vi "U6 Multiple LJTDAC Loop.vi"() -> (0 "error out":errorcluster)   [LabVIEW 2021]
panel:
  in  "Interval (ms)":u32=500
  in  "stop":bool
  in  "2nd DACB":dbl step=0.1 format="%.4f"
  in  "2nd DACA":dbl step=0.1 format="%.4f"
  in  "2nd TDAC SCL Pin #":i32=2
  in  "1st DACB":dbl step=0.1 format="%.4f"
  in  "1st DACA":dbl step=0.1 format="%.4f"
  in  "FirstFound":bool=TRUE
  in  "Address":string="1"
  out "Error Message":string
  in  "1st TDAC SCL Pin #":i32
  # "Updates both channels on an LJTick-DAC."
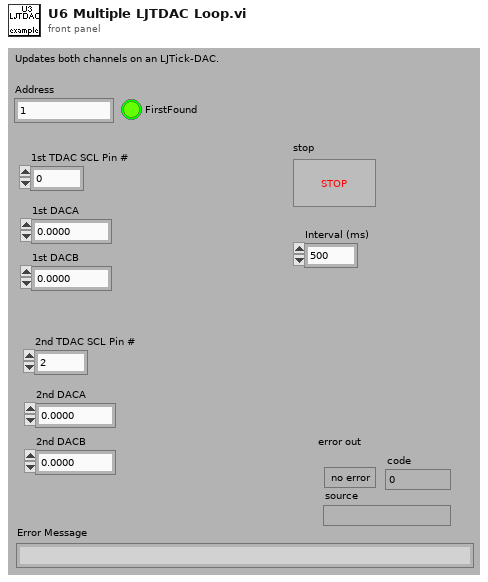
[diagram p1: front panel]
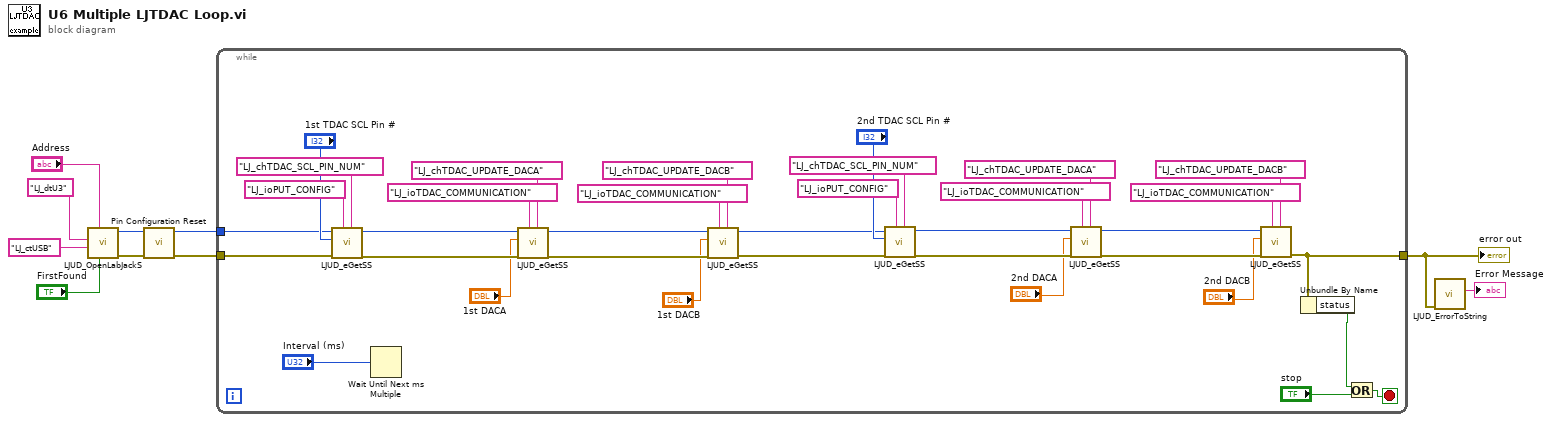
[diagram p0: block diagram]
diagram:
  n1 = call "LJUD_OpenLabJackS.vi"("FirstFound"="FirstFound", "Address"="Address", "ConnectionType"="LJ_ctUSB", "DeviceType"="LJ_dtU3") -> ("error out"=w4:errorcluster, "Handle"=w5:i32)  [unwired: 5 in, 1 out]
  n2 = call "Pin Configuration Reset.vi"("error in"=w4, "Handle In"=w5) -> ("error out"=w2:errorcluster, "Handle Out"=w3:i32)  [unwired: 8 in]
  n3 = while {
    tunnel: w3 -> [w42]
    tunnel: w2 -> [w41]
    tunnel: [w11] -> w1
    stop <- w16 stop-if-true
    n4 = call "LJUD_eGetSS.vi"("Channel"="LJ_chTDAC_SCL_PIN_NUM", "IOType"="LJ_ioPUT_CONFIG", "error in"=w41, "Value Write"="1st TDAC SCL Pin #", "Handle In"=w42) -> ("error out"=w37:errorcluster, "Handle Out"=w38:i32)  [unwired: 4 in, 1 out]
    n5 = Wait Until Next ms Multiple(millisecond multiple="Interval (ms)") -> ()  [unwired: 1 out]
    n6 = call "LJUD_eGetSS.vi"("Channel"="LJ_chTDAC_UPDATE_DACA", "IOType"="LJ_ioTDAC_COMMUNICATION", "error in"=w37, "Value Write"="1st DACA", "Handle In"=w38) -> ("error out"=w32:errorcluster, "Handle Out"=w33:i32)  [unwired: 4 in, 1 out]
    n7 = call "LJUD_eGetSS.vi"("Channel"="LJ_chTDAC_UPDATE_DACB", "IOType"="LJ_ioTDAC_COMMUNICATION", "error in"=w32, "Value Write"="1st DACB", "Handle In"=w33) -> ("error out"=w12:errorcluster, "Handle Out"=w13:i32)  [unwired: 4 in, 1 out]
    n8 = call "LJUD_eGetSS.vi"("Channel"="LJ_chTDAC_SCL_PIN_NUM", "IOType"="LJ_ioPUT_CONFIG", "error in"=w12, "Value Write"="2nd TDAC SCL Pin #", "Handle In"=w13) -> ("error out"=w26:errorcluster, "Handle Out"=w25:i32)  [unwired: 4 in, 1 out]
    n9 = call "LJUD_eGetSS.vi"("Channel"="LJ_chTDAC_UPDATE_DACA", "IOType"="LJ_ioTDAC_COMMUNICATION", "error in"=w26, "Value Write"="2nd DACA", "Handle In"=w25) -> ("error out"=w30:errorcluster, "Handle Out"=w29:i32)  [unwired: 4 in, 1 out]
    n10 = call "LJUD_eGetSS.vi"("Channel"="LJ_chTDAC_UPDATE_DACB", "IOType"="LJ_ioTDAC_COMMUNICATION", "error in"=w30, "Value Write"="2nd DACB", "Handle In"=w29) -> ("error out"=w11:errorcluster)  [unwired: 4 in, 2 out]
    n11 = Unbundle By Name(w11) -> ("status"=w15:bool)
    n12 = Or(x=w15, y="stop") -> (x .or. y?=w16:bool)
  }
  "error out" <- w1
  n13 = call "LJUD_ErrorToString.vi"("error in"=w1) -> ("String"=→"Error Message":string)  [unwired: 10 in]
